vi "pop_number.vi"(8 "error in (no error)":errorcluster, 11 "Lua in":refnum<class "Lua.lvclass">) -> (0 "error out":errorcluster, 2 "value":dbl, 3 "Lua out":refnum<class "Lua.lvclass">)   [LabVIEW 2020, in "Lua for LabVIEW.lvlib" / "Lua.lvclass"]
doc: "Pop a numeric value from the stack."
uses:
  Lua.lvclass
  Lua.lvclass/Lua.ctl
  lib/lua.dll/lua.dll.lvlib
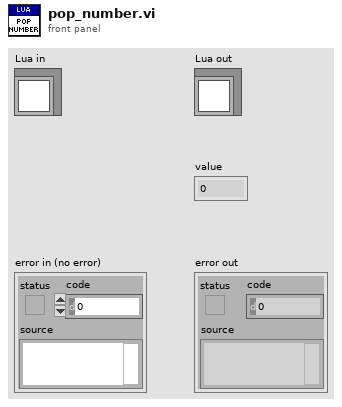
[diagram p1: front panel]
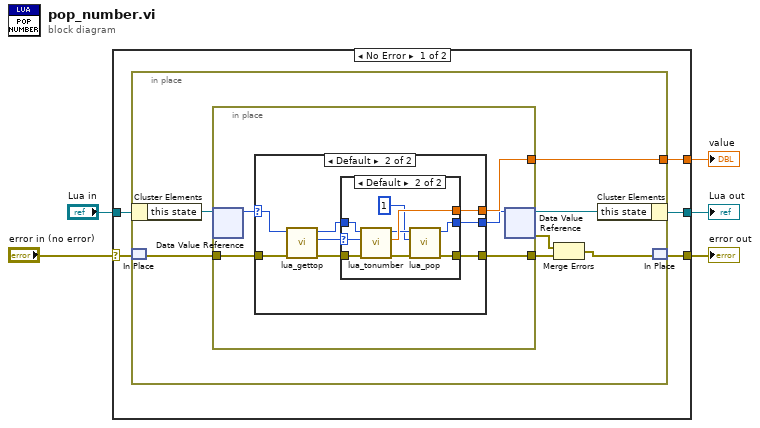
[diagram p0: block diagram]
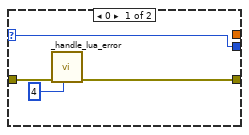
[diagram p2: hidden frame]
diagram:
  n1 = case shown="No Error" "error in (no error)" {
    selector: "error in (no error)" -> [w7 w47]
    tunnel: [w8 w47] -> w4
    tunnel: [w9 w46] -> w2
    tunnel: "Lua in" -> [w10 w46]
    tunnel: [w6 _] -> w1
    frame No Error {
      n2 = in-place {
        in-place-border: [w16] -> w6
        n3 = in-place-cluster #1(w10) -> ("this state"=w15:refnum<data-value>)
        n4 = in-place-match #2(w7) -> (w17:errorcluster)
        n5 = in-place {
          in-place-border: w17 -> [w22]
          in-place-border: [w21] -> w16
          in-place-border: [w18] -> w13
          n6 = in-place-dvr #3(w15) -> (w20:u64)  [unwired: 1 out]
          n7 = case shown="Default" w20 {
            selector: w20 -> [w26 w30]
            tunnel: [w26 w32] -> w19
            tunnel: w22 -> [w23 w31]
            tunnel: [w24 w33] -> w18
            tunnel: [_ w34] -> w21
            frame 0 {
              n8 = call "_handle_lua_error.vi"("lua status"=4 ("lua_load errcode"), "error in (no error)"=w23) -> ("error out"=w24:errorcluster)  [unwired: 9 in]
            }
            frame Default {
              n9 = call "lua_gettop.vi"("error in (no error)"=w31, "lua_state_p"=w30) -> ("error out"=w27:errorcluster, "index"=w29:i32, "lua_state_p out"=w28:u64)  [unwired: 7 in]
              n10 = case shown="Default" w29 {
                selector: w29 -> [_ w38]
                tunnel: [_ w45] -> w34
                tunnel: [w35 w43] -> w33
                tunnel: [w36 w42] -> w32
                tunnel: w28 -> [w36 w39]
                tunnel: w27 -> [w35 w37]
                frame 0 {
                }
                frame Default {
                  n11 = call "lua_tonumber.vi"("error in (no error)"=w37, "index"=w38, "lua_state_p"=w39) -> ("error out"=w44:errorcluster, "number"=w45:dbl, "lua_state_p out"=w41:u64)  [unwired: 5 in, 1 out]
                  n12 = call "lua_pop.vi"("error in (no error)"=w44, "n"=1 ("index"), "lua_state_p"=w41) -> ("error out"=w43:errorcluster, "lua_state_p out"=w42:u64)  [unwired: 7 in]
                }
              }
            }
          }
          n13 = in-place-dvr #3(w19) -> (w14:refnum<data-value>, w12:errorcluster)
        }
        n14 = Merge Errors(w12, w13) -> (w11:errorcluster)
        n15 = in-place-cluster #1("this state"=w14) -> (w9:refnum<class "Lua.lvclass">)
        n16 = in-place-match #2(w11) -> (w8:errorcluster)
      }
    }
    frame Error {
    }
  }
  "error out" <- w4
  "Lua out" <- w2
  "value" <- w1
